vi "KE6221 -- Set Arb Waveform Points.vi"(0 "Resource In":refnum<visa-resource-name>, 1 "Check For SCPI Errors? (T)":bool=TRUE, 5 "Arb Location":T1, 7 "Arb Waveform Points In":T2[](array[typedef]) min=-1.0 max=1.0 format="%.3f", 11 "error in (no error)":errorcluster, 12 "Read Back Set Values? (T)":bool=TRUE, 13 "Timeout (10 s)":u32=10000) -> (4 "Resource Out (dupl)":refnum<visa-resource-name>, 6 "Num Points Out":u32, 8 "Arb Waveform Points Out":T2[](array[typedef]) min=-1.0 max=1.0 format="%.3f", 15 "error out":errorcluster)   [LabVIEW 2019, in "Keithley 622x.lvlib"]
uses:
  Keithley 622x.lvlib
  Typedefs/KE6221 -- Wave Arb Point.ctl
  Typedefs/KE6221 -- Arb Location.ctl
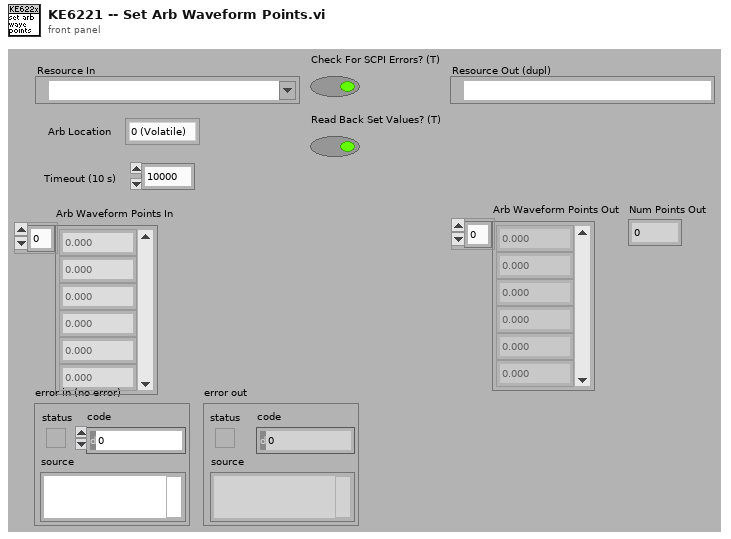
[diagram p1: front panel]
types:
  T1 = typedef "Keithley 622x.lvlib/KE6221 -- Arb Location.ctl" = enum16{"0 (Volatile)", "1 (NVRAM)", "2 (NVRAM)", "3 (NVRAM)", "4 (NVRAM)"}
  T2 = typedef "Keithley 622x.lvlib/KE6221 -- Wave Arb Point.ctl" = dbl
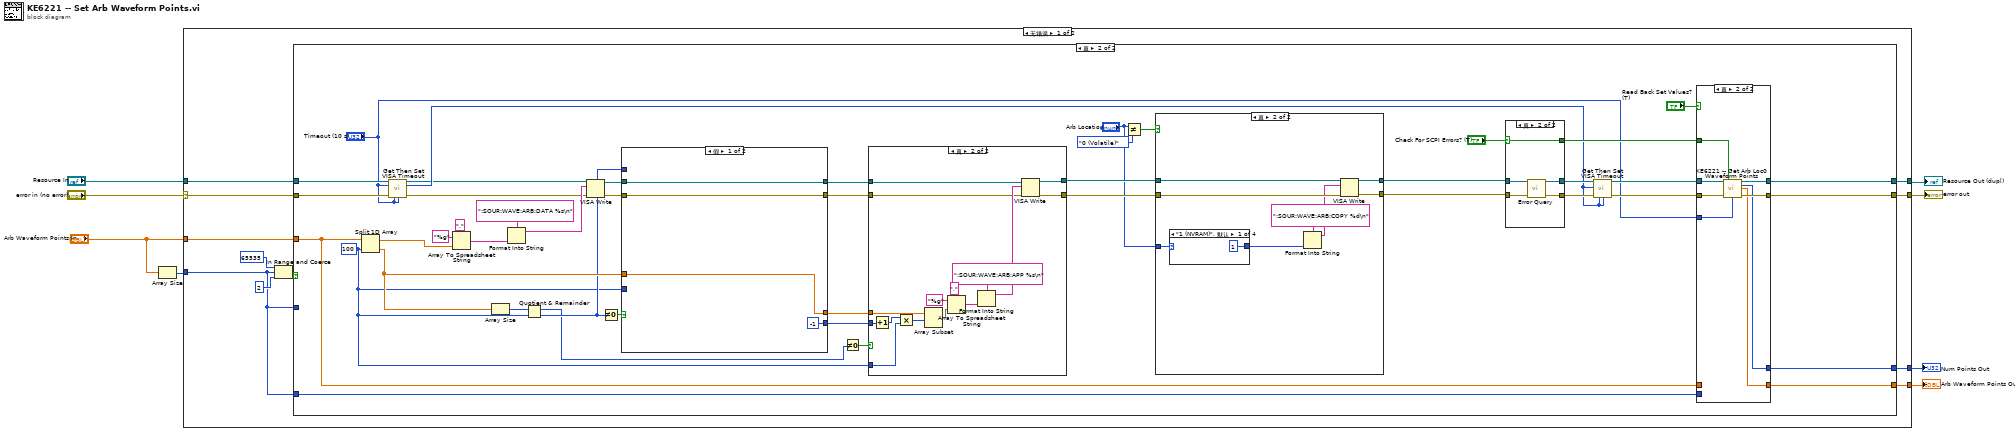
[diagram p0: block diagram]
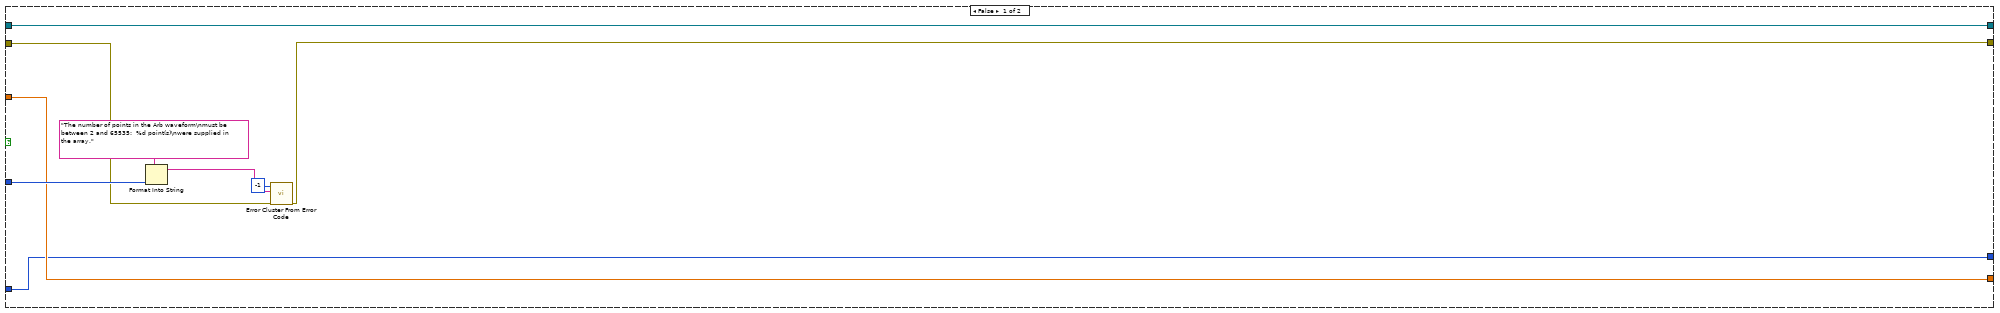
[diagram p2: hidden frame]
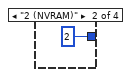
[diagram p4: hidden frame]
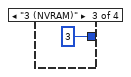
[diagram p5: hidden frame]
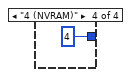
[diagram p6: hidden frame]
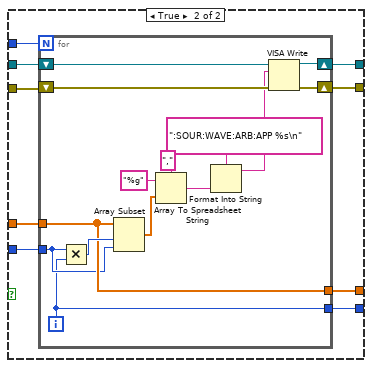
[diagram p10: hidden frame]
diagram:
  n1 = Array Size(array="Arb Waveform Points In") -> (size(s)=w1:i32)
  n2 = case shown="无错误" "error in (no error)" {
    selector: "error in (no error)" -> [w9 w153]
    tunnel: "Resource In" -> [w10 w152]
    tunnel: [w16 w152] -> w4
    tunnel: [w15 w153] -> w3
    tunnel: "Arb Waveform Points In" -> [w14 w154]
    tunnel: [w13 w154] -> w6
    tunnel: [w12 w155] -> w5
    tunnel: w1 -> [w11 w155]
    frame No Error {
      n3 = In Range and Coerce(upper limit=65535, x=w11, lower limit=2) -> (In Range?=w17:bool)  [unwired: 1 out]
      n4 = case shown="真" w17 {
        tunnel: w9 -> [w23 w42]
        tunnel: w11 -> [w27 _]
        tunnel: w14 -> [w21 w51]
        tunnel: w10 -> [w22 w43]
        tunnel: [w22 w35] -> w16
        tunnel: [w24 w34] -> w15
        tunnel: [w20 w50] -> w12
        tunnel: [w21 w49] -> w13
        tunnel: w11 -> [w20 w48]
        frame False {
          n5 = Format Into String(format string="The number of points in the Arb waveform\nmust be between 2 and 65535:  %d point(s)\nwere supplied in the array.", w27) -> (resulting string=w26:string)  [unwired: 2 in, 1 out]
          n6 = call <vilib>:"Error Cluster From Error Code.vi"("error in (no error)"=w23, "error message (\"\")"=w26, "error code (0)"=-1) -> ("error out"=w24:errorcluster)  [unwired: 6 in]
        }
        frame True {
          w58 = 100 ("index")
          n7 = Split 1D Array(array=w51, index=w58) -> (first subarray=w67:T2[], second subarray=w65:T2[])
          n8 = call "Get Then Set VISA Timeout.vi"("VISA Resource Name In"=w43, "New Timeout (msecs)"="Timeout (10 s)", "error in (no error)"=w42, "Max Timeout (300 secs)"="Timeout (10 s)", "Min Timeout (3 secs)"="Timeout (10 s)") -> ("VISA Resource Name Out (dupl)"=w30:refnum<visa-resource-name>, "Old Timeout (msecs)"=w37:u32, "error out"=w29:errorcluster)  [unwired: 7 in, 1 out]
          n9 = Array To Spreadsheet String(delimiter (Tab)=",", array=w67, 3:"%g" ("format string")) -> (spreadsheet string=w70:string)
          n10 = Array Size(array=w65) -> (size(s)=w66:i32)
          n11 = Format Into String(format string=":SOUR:WAVE:ARB:DATA %s\n", w70) -> (resulting string=w69:string)  [unwired: 2 in, 1 out]
          n12 = Quotient & Remainder(x=w66, y=w58) -> (x-y*floor(x/y)=w61:i32, floor(x/y)=w64:i32)
          n13 = VISA Write(VISA resource name=w30, write buffer=w69, error in (no error)=w29) -> (VISA resource name out=w63:refnum<visa-resource-name>, error out=w62:errorcluster)  [unwired: 1 out]
          n14 = Not Equal To 0?(x=w64) -> (x != 0?=w68:bool)
          n15 = case shown="假" w68 {
            tunnel: w65 -> [w126 w137]
            tunnel: w64 -> [_ w136]
            tunnel: w58 -> [_ w135]
            tunnel: w63 -> [w128 w134]
            tunnel: w62 -> [w127 w133]
            tunnel: [w126 w132] -> w57
            tunnel: [-1 w131] -> w59
            tunnel: [w127 w130] -> w56
            tunnel: [w128 w129] -> w55
            frame False {
            }
            frame True {
              n16 = for {
                N: w136 -> [_]
                tunnel: w137 -> [w140]
                tunnel: w135 -> [w139]
                shift-right: [w142] -> w129
                shift-left: w134 -> [w143]
                shift-right: [w141] -> w130
                shift-left: w133 -> [w145]
                tunnel: [w140] -> w132
                tunnel: [w138] -> w131
                i -> [w138]
                n17 = Multiply(x=w139, y=w138) -> (x*y=w151:i32)
                n18 = Array Subset(array=w140, index=w151, length=w139) -> (w146:T2[])
                n19 = Array To Spreadsheet String(delimiter (Tab)=",", array=w146, 3:"%g" ("format string")) -> (spreadsheet string=w150:string)
                n20 = Format Into String(format string=":SOUR:WAVE:ARB:APP %s\n", w150) -> (resulting string=w144:string)  [unwired: 2 in, 1 out]
                n21 = VISA Write(VISA resource name=w143, write buffer=w144, error in (no error)=w145) -> (VISA resource name out=w142:refnum<visa-resource-name>, error out=w141:errorcluster)  [unwired: 1 out]
              }
            }
          }
          n22 = Not Equal To 0?(x=w61) -> (x != 0?=w60:bool)
          n23 = case shown="真" w60 {
            tunnel: w59 -> [_ w124]
            tunnel: w58 -> [_ w122]
            tunnel: w57 -> [_ w120]
            tunnel: w56 -> [w108 w113]
            tunnel: w55 -> [w109 w112]
            tunnel: [w108 w111] -> w46
            tunnel: [w109 w110] -> w47
            frame False {
            }
            frame True {
              n24 = Increment(x=w124) -> (x+1=w123:i32)
              n25 = Multiply(x=w123, y=w122) -> (x*y=w121:i32)
              n26 = Array Subset(array=w120, index=w121) -> (w115:T2[])  [unwired: 1 in]
              n27 = Array To Spreadsheet String(delimiter (Tab)=",", array=w115, 3:"%g" ("format string")) -> (spreadsheet string=w114:string)
              n28 = Format Into String(format string=":SOUR:WAVE:ARB:APP %s\n", w114) -> (resulting string=w119:string)  [unwired: 2 in, 1 out]
              n29 = VISA Write(VISA resource name=w112, write buffer=w119, error in (no error)=w113) -> (VISA resource name out=w110:refnum<visa-resource-name>, error out=w111:errorcluster)  [unwired: 1 out]
            }
          }
          n30 = Not Equal?(x="Arb Location", y=KE6221_--_Arb_Location."0 (Volatile)") -> (x != y?=w32:bool)
          n31 = case shown="真" w32 {
            tunnel: w47 -> [w75 w82]
            tunnel: w46 -> [w74 w81]
            tunnel: [w74 w79] -> w44
            tunnel: [w75 w78] -> w45
            tunnel: "Arb Location" -> [_ w77]
            frame False {
            }
            frame True {
              n32 = case shown="\"1 (NVRAM)\", 默认" w77 {
                tunnel: [1 2 3 4] -> w76
                frame "1 (NVRAM)", Default {
                }
                frame "2 (NVRAM)" {
                }
                frame "3 (NVRAM)" {
                }
                frame "4 (NVRAM)" {
                }
              }
              n33 = Format Into String(format string=":SOUR:WAVE:ARB:COPY %d\n", w76) -> (resulting string=w80:string)  [unwired: 2 in, 1 out]
              n34 = VISA Write(VISA resource name=w82, write buffer=w80, error in (no error)=w81) -> (VISA resource name out=w78:refnum<visa-resource-name>, error out=w79:errorcluster)  [unwired: 1 out]
            }
          }
          n35 = case shown="真" "Check For SCPI Errors? (T)" {
            selector: "Check For SCPI Errors? (T)" -> [w100 w103]
            tunnel: w45 -> [w102 w107]
            tunnel: w44 -> [w101 w106]
            tunnel: [w101 w105] -> w40
            tunnel: [w102 w104] -> w41
            tunnel: [w100 w103] -> w54
            frame False {
            }
            frame True {
              n36 = call "Error Query.vi"("VISA Resource In"=w107, "error in (no error)"=w106) -> ("VISA Resource Out (dupl)"=w104:refnum<visa-resource-name>, "error out"=w105:errorcluster)  [unwired: 10 in, 2 out]
            }
          }
          n37 = call "Get Then Set VISA Timeout.vi"("VISA Resource Name In"=w41, "New Timeout (msecs)"=w37, "error in (no error)"=w40, "Max Timeout (300 secs)"=w37, "Min Timeout (3 secs)"=w37) -> ("VISA Resource Name Out (dupl)"=w38:refnum<visa-resource-name>, "error out"=w39:errorcluster)  [unwired: 7 in, 2 out]
          n38 = case shown="真" "Read Back Set Values? (T)" {
            tunnel: w38 -> [w91 w99]
            tunnel: w54 -> [_ w98]
            tunnel: w39 -> [w90 w97]
            tunnel: [w91 w96] -> w35
            tunnel: [w90 w95] -> w34
            tunnel: w51 -> [w89 _]
            tunnel: [w89 w94] -> w49
            tunnel: [w88 w93] -> w50
            tunnel: w48 -> [w88 _]
            tunnel: "Timeout (10 s)" -> [_ w92]
            frame False {
            }
            frame True {
              n39 = call "KE6221 -- Get Arb Loc0 Waveform Points.vi"("Resource In"=w99, "Check For SCPI Errors? (T)"=w98, "error in (no error)"=w97, "Timeout (10000 ms)"=w92) -> ("Resource Out (dupl)"=w96:refnum<visa-resource-name>, "Num Points"=w93:u32, "Arb Waveform Points"=w94:T2[], "error out"=w95:errorcluster)  [unwired: 8 in]
            }
          }
        }
      }
    }
    frame Error {
    }
  }
  "Arb Waveform Points Out" <- w6
  "Resource Out (dupl)" <- w4
  "error out" <- w3
  "Num Points Out" <- w5
